vi "SVT Shock Response Spectrum.vi"   [LabVIEW 2017, in "SoundVib_Transient.lvlib"]
doc: "Computes the peak levels for each single-degree-of-freedom (SDOF) component to form the shock response spectrum (SRS) across the <B>frequency range</B> of interest. Wire data to the <B>scaled signal [EU]</B> input to determine the polymorphic instance to use or manually select the instance."
uses:
  <vilib>/addons/Sound and Vibration/svt_Transients/SoundVib_Transient.lvlib
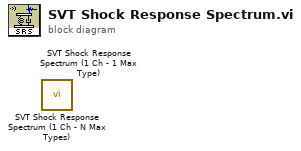
[diagram p0: block diagram]
diagram:
  n1 = call <vilib>:"SVT Shock Response Spectrum (1 Ch - N Max Types).vi"() -> ()  [unwired: 13 in, 3 out]
  n2 = call <vilib>:"SVT Shock Response Spectrum (1 Ch - 1 Max Type).vi"() -> ()  [unwired: 13 in, 3 out]
